vi "Conditional Increment - I32.vi"(2 "Condition":bool, 3 "Input":i32) -> (0 "Output":i32)   [LabVIEW 2012, in "femtoRoboLib.lvlib"]
uses:
  femtoRoboLib.lvlib
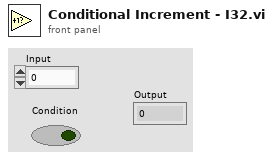
[diagram p1: front panel]
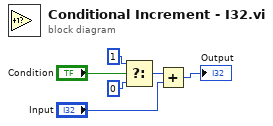
[diagram p0: block diagram]
diagram:
  n1 = Select(t=1, s="Condition", f=0 ("t")) -> (s? t:f=w4:i32)
  n2 = Add(x=w4, y="Input") -> (x+y=→"Output":i32)
